vi "SP Delete Marker from Plots.vi"(7 "Plot References":refnum<vi>[](array[refnum]), 8 "error in (no error)":errorcluster, 9 "Deleted Marker":i8, 10 "Marker Table":refnum<vi>, 11 "Plot Ref":refnum<vi>) -> (0 "error out":errorcluster)   [LabVIEW 2011]
uses:
  TypeDefs/SP Plot Cluster Object.ctl
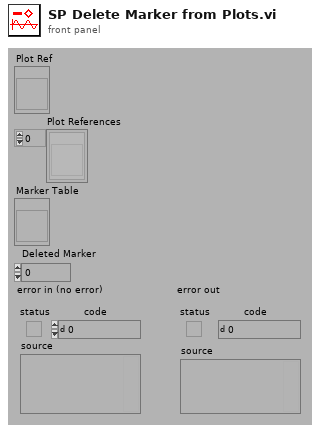
[diagram p1: front panel]
types:
  T1 = typedef "SP Plot Cluster Object.ctl" = enum16{"Plot", "CH Reference", "CH Label", "Start Label", "Stop Label", "Units Label", "Selected?", "CH Markers"}
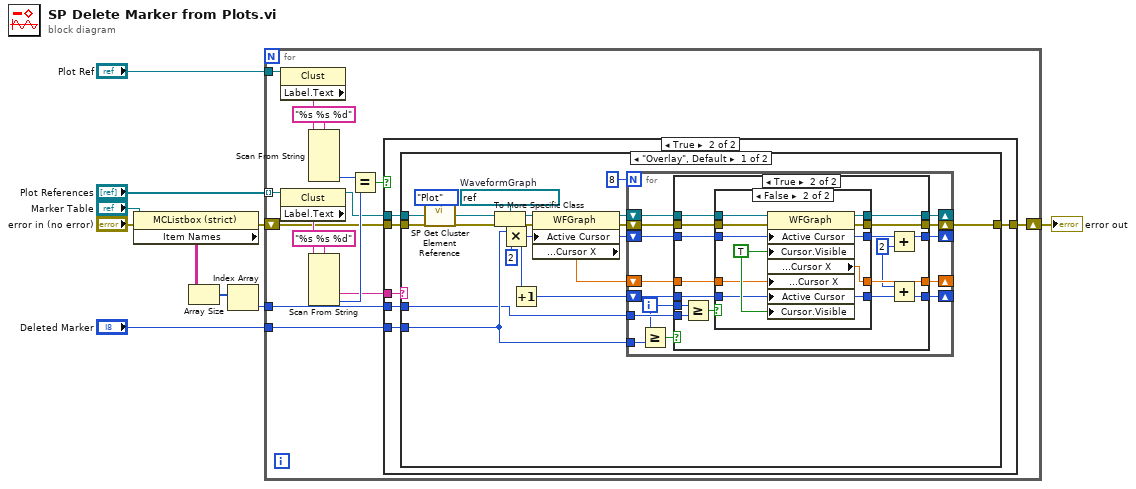
[diagram p0: block diagram]
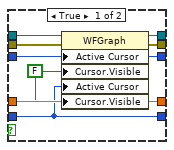
[diagram p4: hidden frame]
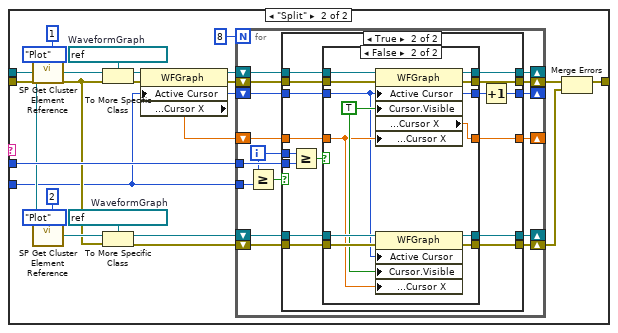
[diagram p5: hidden frame]
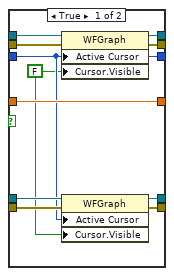
[diagram p7: hidden frame]
diagram:
  n1 = property class="MCListbox (strict)"(reference="Marker Table", error in="error in (no error)") -> (error out=w8:errorcluster, "Item Names"=w6:string[][])  [unwired: 1 out]
  n2 = Array Size(array=w6) -> (size(s)=w5:i32[])
  n3 = Index Array(array=w5) -> (element=w3:i32)  [unwired: 1 in]
  n4 = for {
    tunnel: "Deleted Marker" -> [w24]
    tunnel: w3 -> [w23]
    tunnel: "Plot References" -> [w13] mode=indexing
    tunnel: "Plot Ref" -> [w11]
    shift-right: [w25] -> w7
    shift-left: w8 -> [w16]
    n5 = property class="Clust"(reference=w11) -> ("Label.Text"=w20:string)  [unwired: 1 in, 2 out]
    n6 = property class="Clust"(reference=w13) -> (reference out=w12:refnum<vi>, "Label.Text"=w18:string)  [unwired: 1 in, 1 out]
    n7 = Scan From String(format string="%s %s %d", input string=w20) -> (output 3=w21:i32)  [unwired: 2 in, 8 out]
    n8 = Scan From String(format string="%s %s %d", input string=w18) -> (output 2=w14:string, output 3=w22:i32)  [unwired: 2 in, 7 out]
    n9 = Equal?(x=w21, y=w22) -> (x = y?=w15:bool)
    n10 = case shown="True" w15 {
      tunnel: w16 -> [w26 w32]
      tunnel: [w26 w31] -> w25
      tunnel: w24 -> [_ w30]
      tunnel: w23 -> [_ w29]
      tunnel: w12 -> [_ w28]
      tunnel: w14 -> [_ w27]
      frame False {
      }
      frame True {
        n11 = case shown="\"Overlay\", Default" w27 {
          tunnel: w32 -> [w48 w108]
          tunnel: [w47 w101] -> w31
          tunnel: w30 -> [w46 w104]
          tunnel: w29 -> [w34 w115]
          tunnel: w28 -> [w33 w109]
          frame "Overlay", Default {
            w43 = refnum<vi> refnum  # WaveformGraph
            n12 = call "SP Get Cluster Element Reference.vi"("Element"=SP_Plot_Cluster_Object."Plot", "Plot Reference"=w33) -> ("Element Reference"=w44:refnum<vi>)  [unwired: 1 in, 6 out]
            n13 = To More Specific Class(target class=w43, reference=w44) -> (specific class reference=w39:refnum<vi>)  [unwired: 1 in, 1 out]
            n14 = Multiply(x=w46, y=2) -> (x*y=w38:i32)
            n15 = Increment(x=w38) -> (x+1=w40:i32)
            n16 = property class="WFGraph"(reference=w39, error in=w48, "Active Cursor"=w38) -> (reference out=w36:refnum<vi>, error out=w35:errorcluster, "Cursor.Cursor Position:Cursor X"=w37:dbl)
            n17 = for {
              N: 8 -> [_]
              shift-right: [w60] -> w47
              shift-left: w35 -> [w59]
              shift-right: [w61] -> _
              shift-left: w36 -> [w62]
              tunnel: w46 -> [w57]
              shift-right: [w55] -> _
              shift-left: w37 -> [w54]
              shift-right: [w52] -> _
              shift-left: w40 -> [w51]
              shift-right: [w53] -> _
              shift-left: w38 -> [w56]
              tunnel: w34 -> [w50]
              i -> [w49]
              n18 = Greater Or Equal?(x=w49, y=w57) -> (x >= y?=w58:bool)
              n19 = case shown="True" w58 {
                tunnel: w62 -> [w67 w83]
                tunnel: [w67 w82] -> w61
                tunnel: [w66 w81] -> w60
                tunnel: w59 -> [w66 w80]
                tunnel: w56 -> [w65 w78]
                tunnel: [w64 w77] -> w55
                tunnel: w54 -> [w64 w76]
                tunnel: [w63 w72] -> w52
                tunnel: [w65 w71] -> w53
                tunnel: w51 -> [w63 w70]
                tunnel: w49 -> [_ w69]
                tunnel: w50 -> [_ w68]
                frame False {
                }
                frame True {
                  w73 = 2 ("y")
                  n20 = Greater Or Equal?(x=w69, y=w68) -> (x >= y?=w79:bool)
                  n21 = case shown="False" w79 {
                    tunnel: w83 -> [w91 w100]
                    tunnel: [w90 w99] -> w82
                    tunnel: [w89 w98] -> w81
                    tunnel: w80 -> [w88 w97]
                    tunnel: w78 -> [w87 w92]
                    tunnel: [w86 w96] -> w77
                    tunnel: w76 -> [w86 w94]
                    tunnel: [w87 w92] -> w75
                    tunnel: [w85 w93] -> w74
                    tunnel: w70 -> [w85 w93]
                    frame True {
                      w84 = FALSE ("Cursor.Visible")
                      n22 = property class="WFGraph"(reference=w91, error in=w88, "Active Cursor"=w87, "Cursor.Visible"=w84, "Active Cursor"=w85, "Cursor.Visible"=w84) -> (reference out=w90:refnum<vi>, error out=w89:errorcluster)
                    }
                    frame False {
                      w95 = TRUE ("Cursor.Visible")
                      n23 = property class="WFGraph"(reference=w100, error in=w97, "Active Cursor"=w92, "Cursor.Visible"=w95, "Cursor.Cursor Position:Cursor X"=w94, "Active Cursor"=w93, "Cursor.Visible"=w95) -> (reference out=w99:refnum<vi>, error out=w98:errorcluster, "Cursor.Cursor Position:Cursor X"=w96:dbl)
                    }
                  }
                  n24 = Add(x=w75, y=w73) -> (x+y=w71:i32)
                  n25 = Add(x=w73, y=w74) -> (x+y=w72:i32)
                }
              }
            }
          }
          frame "Split" {
            w112 = refnum<vi> refnum  # WaveformGraph
            w121 = refnum<vi> refnum  # WaveformGraph
            n26 = call "SP Get Cluster Element Reference.vi"("Channel"=i8 1, "Element"=SP_Plot_Cluster_Object."Plot", "Plot Reference"=w109) -> ("Element Reference"=w122:refnum<vi>)  [unwired: 6 out]
            n27 = call "SP Get Cluster Element Reference.vi"("Channel"=i8 2, "Element"=SP_Plot_Cluster_Object."Plot", "Plot Reference"=w109) -> ("Element Reference"=w111:refnum<vi>)  [unwired: 6 out]
            n28 = To More Specific Class(target class=w121, reference=w122, error in=w108) -> (specific class reference=w119:refnum<vi>, error out=w107:errorcluster)
            n29 = To More Specific Class(target class=w112, reference=w111, error in=w108) -> (specific class reference=w106:refnum<vi>, error out=w105:errorcluster)
            n30 = property class="WFGraph"(reference=w119, error in=w107, "Active Cursor"=w104) -> (reference out=w117:refnum<vi>, error out=w116:errorcluster, "Cursor.Cursor Position:Cursor X"=w118:dbl)
            n31 = for {
              N: 8 -> [_]
              shift-right: [w137] -> w102
              shift-left: w116 -> [w136]
              shift-right: [w138] -> _
              shift-left: w117 -> [w139]
              tunnel: w104 -> [w134]
              shift-right: [w132] -> _
              shift-left: w118 -> [w131]
              shift-right: [w130] -> _
              shift-left: w104 -> [w133]
              tunnel: w115 -> [w129]
              shift-right: [w125] -> w103
              shift-left: w105 -> [w126]
              shift-right: [w124] -> _
              shift-left: w106 -> [w127]
              i -> [w128]
              n32 = Greater Or Equal?(x=w128, y=w134) -> (x >= y?=w135:bool)
              n33 = case shown="True" w135 {
                tunnel: w139 -> [w145 w161]
                tunnel: [w145 w160] -> w138
                tunnel: [w144 w159] -> w137
                tunnel: w136 -> [w144 w158]
                tunnel: w133 -> [w143 w156]
                tunnel: [w142 w155] -> w132
                tunnel: w131 -> [w142 w154]
                tunnel: [w143 w153] -> w130
                tunnel: w128 -> [_ w152]
                tunnel: w129 -> [_ w151]
                tunnel: w127 -> [w141 w149]
                tunnel: w126 -> [w140 w148]
                tunnel: [w140 w147] -> w125
                tunnel: [w141 w146] -> w124
                frame False {
                }
                frame True {
                  n34 = Greater Or Equal?(x=w152, y=w151) -> (x >= y?=w157:bool)
                  n35 = case shown="False" w157 {
                    tunnel: w161 -> [w172 w184]
                    tunnel: [w171 w183] -> w160
                    tunnel: [w170 w182] -> w159
                    tunnel: w158 -> [w169 w181]
                    tunnel: w156 -> [w163 w173]
                    tunnel: [w168 w180] -> w155
                    tunnel: w154 -> [w168 w176]
                    tunnel: [w163 w173] -> w150
                    tunnel: w149 -> [w167 w178]
                    tunnel: w148 -> [w164 w179]
                    tunnel: [w165 w175] -> w147
                    tunnel: [w166 w174] -> w146
                    frame True {
                      w162 = FALSE ("Cursor.Visible")
                      n36 = property class="WFGraph"(reference=w172, error in=w169, "Active Cursor"=w163, "Cursor.Visible"=w162) -> (reference out=w171:refnum<vi>, error out=w170:errorcluster)
                      n37 = property class="WFGraph"(reference=w167, error in=w164, "Active Cursor"=w163, "Cursor.Visible"=w162) -> (reference out=w166:refnum<vi>, error out=w165:errorcluster)
                    }
                    frame False {
                      w177 = TRUE ("Cursor.Visible")
                      n38 = property class="WFGraph"(reference=w184, error in=w181, "Active Cursor"=w173, "Cursor.Visible"=w177, "Cursor.Cursor Position:Cursor X"=w176) -> (reference out=w183:refnum<vi>, error out=w182:errorcluster, "Cursor.Cursor Position:Cursor X"=w180:dbl)
                      n39 = property class="WFGraph"(reference=w178, error in=w179, "Active Cursor"=w173, "Cursor.Visible"=w177, "Cursor.Cursor Position:Cursor X"=w176) -> (reference out=w174:refnum<vi>, error out=w175:errorcluster)
                    }
                  }
                  n40 = Increment(x=w150) -> (x+1=w153:i8)
                }
              }
            }
            n41 = Merge Errors(w102, w103) -> (w101:errorcluster)
          }
        }
      }
    }
  }
  "error out" <- w7
